vi "Gateway_Connect.vi"(8 "error in (no error)":errorcluster, 11 "GatewayClass in":refnum<class "GatewayClass.lvclass">) -> (0 "error out":errorcluster, 2 "MIDAS Forwarding Address":string, 3 "GatewayClass out":refnum<class "GatewayClass.lvclass">)   [LabVIEW 2018, in "feGEM Gateway.lvlib" / "GatewayClass.lvclass"]
uses:
  GatewayClass.lvclass
  GatewayClass.lvclass/GatewayClass.ctl
  DataPacker/Utilities/SSH_TUNNEL.lvclass
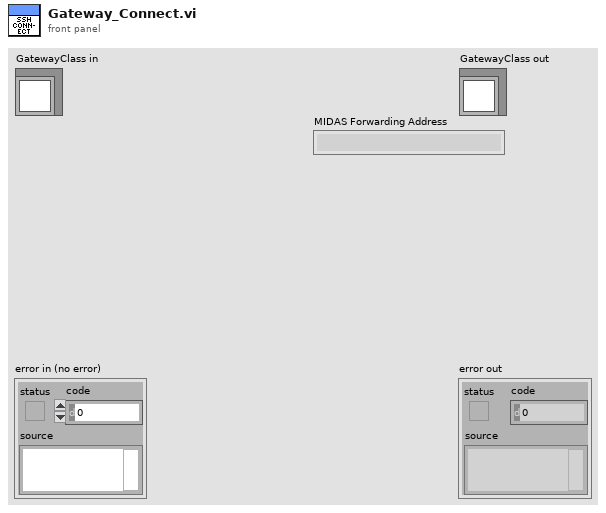
[diagram p1: front panel]
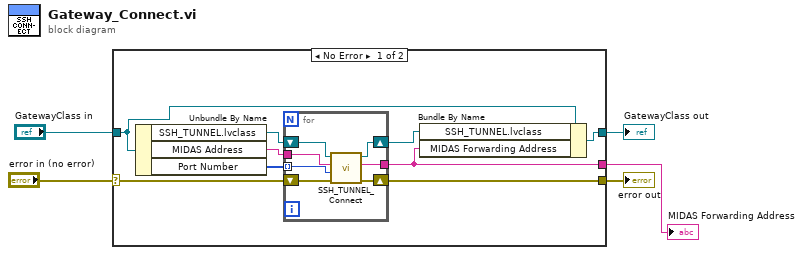
[diagram p0: block diagram]
diagram:
  n1 = case shown="No Error" "error in (no error)" {
    selector: "error in (no error)" -> [w13 w23]
    tunnel: [w10 w23] -> w4
    tunnel: [w11 w22] -> w2
    tunnel: "GatewayClass in" -> [w12 w22]
    tunnel: [w7 _] -> w1
    frame No Error {
      n2 = Unbundle By Name(w12) -> ("SSH_TUNNEL.lvclass"=w14:refnum<class "SSH_TUNNEL.lvclass">, "MIDAS Address"=w9:string, "Port Number"=w8:u16[])
      n3 = for {
        shift-right: [w19] -> w10
        shift-left: w13 -> [w21]
        tunnel: w9 -> [w17]
        tunnel: w8 -> [w16] mode=indexing
        tunnel: [w15] -> w7
        shift-right: [w20] -> w6
        shift-left: w14 -> [w18]
        n4 = call "SSH_TUNNEL_Connect.vi"("error in (no error)"=w21, "MIDAS Port Number"=w16, "MIDAS Address"=w17, "SSH_TUNNEL in"=w18) -> ("error out"=w19:errorcluster, "MIDAS Address"=w15:string, "SSH_TUNNEL out"=w20:refnum<class "SSH_TUNNEL.lvclass">)  [unwired: 5 in]
      }
      n5 = Bundle By Name(cluster=w12, "SSH_TUNNEL.lvclass"=w6, "MIDAS Forwarding Address"=w7) -> (w11:refnum<class "GatewayClass.lvclass">)
    }
    frame Error {
    }
  }
  "error out" <- w4
  "GatewayClass out" <- w2
  "MIDAS Forwarding Address" <- w1
